vi "Binary Inverse.vi"(8 "error in (no error)":errorcluster, 10 "Image Dst":T1, 11 "Image In":T1) -> (0 "error out":errorcluster, 3 "Image Out":T1)   [LabVIEW 2011]
doc: "Inverts the pixel intensities of a binary image containing two different grayscale intensities in order to compute the negative of an image."
uses:
  <vilib>/vision/Image Controls.llb/IMAQ Image.ctl
  <vilib>/vision/NI_Vision_Development_Module.lvlib
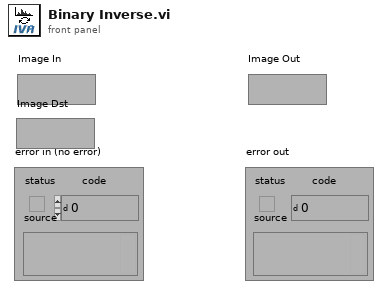
[diagram p1: front panel]
types:
  T1 = typedef "IMAQ Image.ctl" = refnum<image>
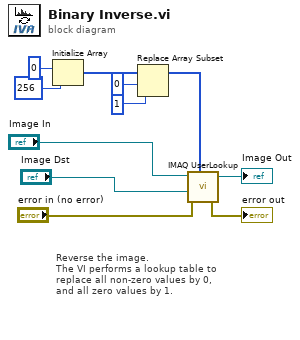
[diagram p0: block diagram]
diagram:
  # "Reverse the image.\nThe VI performs a lookup table to\nreplace all non-zero values by 0,\nand all zero values by 1."
  n1 = Initialize Array(i16 0 ("Element Data"), 256 ("Dimension Size")) -> (w7:i16[])
  n2 = Replace Array Subset(array=w7, new element=i16 1 ("New Element/Subarray"), index=0 ("Index")) -> (w6:i16[])
  n3 = call "IMAQ UserLookup"("Image Src"="Image In", "Lookup Table"=w6, "Image Dst"="Image Dst", "error in (no error)"="error in (no error)") -> ("Image Dst Out"=→"Image Out":T1, "error out"=→"error out":errorcluster)  [unwired: 1 in, 2 out]
